vi "Dashboard Main.vi"() -> ()   [LabVIEW 2015]
uses:
  <vilib>/Utility/miscctls.llb/LVRowAndColumnTypeDef.ctl
  <vilib>/event_ctls.llb/eventvkey.ctl
  <vilib>/Rock Robotics/Network Tables/NT Read Boolean.vi
  <vilib>/Rock Robotics/WPI/Dashboard/WPI_DashboardLogging Global.vi
  <vilib>/Rock Robotics/Network Tables/NT Read Numeric Array.vi
  <vilib>/Utility/config.llb/Write Key (String).vi
  <vilib>/Utility/config.llb/Write Key (I32).vi
  <vilib>/Utility/config.llb/NI_LVConfig.lvlib
  <vilib>/vision/NI_Vision_Development_Module.lvlib
panel:
  in  "TCP":refnum<k5>
  in  "Rec Mode":enum32{"Stop", "Record", "Playback"}(radio)
  in  "Vision":u16(ring) items=["Camera Off", "USB Camera SW", "USB Camera HW", "IP Camera"]
  out "Camera IP":string
  out "Image Message":string="Timeout in Camera Communications"
  in  "Dashboard Tab":T1(tab)
  out "Camera Reversed":bool
  out "dist":dbl
  in  "Select Auto":string(combo)
  out "NT Connection":bool
  in  "Camera Settings":T2={"Frame Rate"=30, "Compression"=30, "Size"=1} {"Frame Rate" scale=1.0..30.0; "Size" items=["640x480", "320x240", "160x120"]}
  out "MotorChart R":cluster{"Numeric":dbl, "Numeric":dbl}(graph)
  out "MotorChart L":T3(graph)
  out "MotorSliders R":cluster{"MotorSlide1":dbl, "MotorSlide2":dbl} {"MotorSlide2" scale=-1.0..1.0 scale format="%#_2e"; "MotorSlide1" scale=-1.0..1.0 scale format="%#_2e"}
  out "MotorSliders L":T4 {"MotorSlide4 2" scale=0.0..14.0 scale format="%#_2e"; "MotorSlide2" scale=-1.0..1.0 scale format="%#_2e"; "MotorSlide1" scale=-1.0..1.0 scale format="%#_2e"}
  out "Gyro":dbl(knob) scale=0.0..360.0
  out "JS1 Z":dbl(slide) scale=-1.0..1.0 scale format="%#_2e"
  out "JS1 Graph":cluster{"X":dbl, "Y":dbl}[](graph)
  out "JS1 Buttons":T5
  out "JS2 Z":dbl(slide) scale=-1.0..1.0 scale format="%#_2e"
  out "JS2 Graph":cluster{"X":dbl, "Y":dbl}[](graph)
  out "JS2 Buttons":T5
  out "Mode":T6(ring)=enum."Auto Disabled"
  in  "DB Camera Config":bool
  out "fps":dbl format="%#.1g"
  out "Mbps":dbl format="%#.1g"
  out "Mbps LED":bool
  in  "DB/String 9":string
  in  "DB/String 8":string
  in  "DB/String 7":string
  in  "DB/String 6":string
  in  "DB/String 5":string
  in  "DB/String 4":string
  in  "DB/String 3":string
  in  "DB/String 2":string
  in  "DB/String 1":string
  in  "DB/String 0":string
  in  "DB/Slider 0":dbl(slide) scale=0.0..5.0
  in  "DB/Slider 1":dbl(slide) scale=0.0..5.0
  in  "DB/Slider 2":dbl(slide) scale=0.0..5.0
  in  "DB/Slider 3":dbl(slide) scale=0.0..5.0
  out "DB/LED 3":bool
  out "DB/LED 2":bool
  out "DB/LED 1":bool
  out "DB/LED 0":bool
  in  "DB/Button 3":bool
  in  "DB/Button 2":bool
  in  "DB/Button 1":bool
  in  "DB/Button 0":bool caption="New Name"
  in  "Test Slider":dbl(slide) scale=0.0..100.0 scale format="%#_3g"
  in  "On/Off":bool caption="Solenoid"
  in  "Test Name":u16(ring) items=["Select the test to run..."]
  in  "Test Tree":string(tree)
  in  "Motor":cluster{"Value":dbl, "Enable":bool} {"Value" scale=-1.0..1.0 scale format="%#_3g"}
  out "Progress":T7 {"Test Progress" scale=0.0..100.0}
  in  "Rev/Fwd":cluster{"Forward":bool, "Reverse":bool}
  in  "Test Ring":u16(ring) items=["Monochrome", "Color"]
  out "Cmd Status":string
  in  "Execute Command":bool
  in  "Command Params":string[][](table)
  in  "Command Selection":i32(listbox)
  in  "CheckList":i32(listbox)
  out "Tree":string(tree)
  out "Camera Image":T8(plugin-control)
  out "Background":bool
  # "Left"
  # "Front"
  # "Right"
  # "Battery"
  # "This tab is a great place for autonomous settings and robot-specific values.\nPlace controls and indicators inside this tab and match name to\nDashboard Variables on robot. You can also delete this comment."
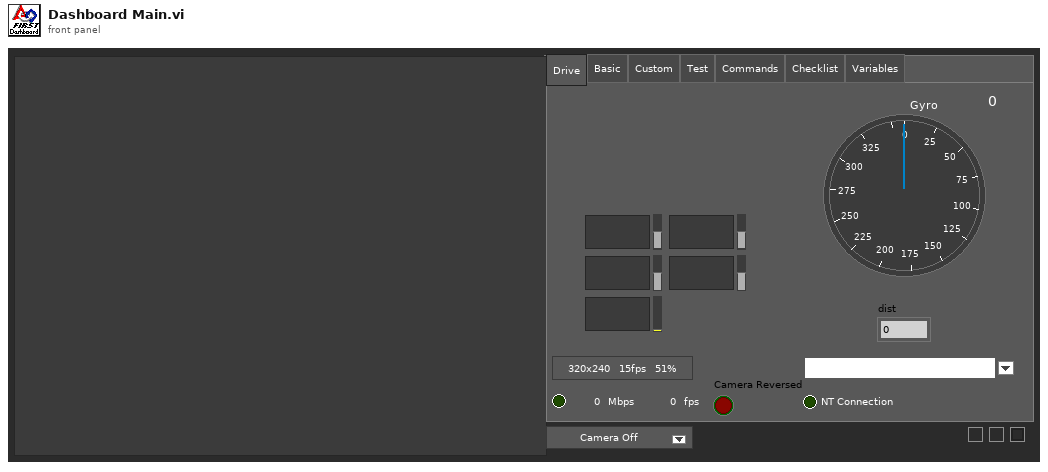
[diagram p1: front panel]
types:
  T1 = enum32{"Drive", "Basic", "Custom", "Test", "Commands", "Checklist", "Variables"}
  T2 = cluster{"Frame Rate":i32, "Compression":i32, "Size":u16}
  T3 = cluster{"Numeric":dbl, "Numeric":dbl, "Battery V":dbl}
  T4 = cluster{"MotorSlide1":dbl, "MotorSlide2":dbl, "MotorSlide4 2":dbl}
  T5 = cluster{bool, bool, bool, bool, bool, bool, bool, bool, bool, bool, bool, bool}
  T6 = enum8{"Tele-Op Disabled", "Tele-Op Enabled", "Auto Disabled", "Auto Enabled", "Test Disabled", "Test Enabled", "Disconnected", "No Code", "E-Stop"}
  T7 = cluster{"Test Progress":u8, "Test Progress Text":string}
  T8 = typedef "IMAQ Image.ctl" = refnum<image>
  T9 = cluster{"IDs":cluster{"RPC field ID":u16, "Unique ID":u16}, "String":string}
  T10 = enum32{"Drive", "Basic", "Custom", "Test", "Checklist", "Variables"}
  T11 = typedef "Image Type" = u32
  T12 = cluster{"Camera Image":refnum<vi>, "Dashboard Tab":refnum<vi>, "Background":refnum<vi>, "Vision":refnum<vi>, "Rec Mode":refnum<vi>, "Test Slider":refnum<vi>, "On/Off ":refnum<vi>, "Test Ring":refnum<vi>, "Rev/Fwd":refnum<vi>, "Test Name":refnum<vi>, "Motor":refnum<vi>, "Progress":refnum<vi>, "CheckList":refnum<vi>, "Tree":refnum<vi>, "Test Tree":refnum<vi>, "Command Params":refnum<vi>, "Command Selection":refnum<vi>, "Execute Command":refnum<vi>, "Cmd Status":refnum<vi>}
  T13 = cluster{"Error Strings":string, "Disable Counts":cluster{u16, u16}, "Rail Faults":cluster{u16, u16, u16}, "Robot IP":string, "DB Mode":u8, "Event Info":cluster{"Name":string, "Type":u8, "Number":u16, "Replay":u8}, "Camera Addr":string}
  T14 = cluster{"Storage":cluster{"Disk Free":u64, "RAM Block":u32, "RAM free":u32}, "CPU Utilization":cluster{"CPU % ISR":sgl, "CPU % Time Crit":sgl, "CPU % Timed Str":sgl, "CPU % High":sgl, "CPU % Above":sgl, "CPU % Normal":sgl, "CPU % Low":sgl}, "CAN":cluster{"% Bus Utilization":sgl, "Bus Off Cnt":u32, "TX_FIFO Full Cnt":u32, "Receive Error Cnt":u8, "Transmit Error Cnt":u8}, "HID":cluster{"HID Outputs":u32, "Rumble Low":u16, "Rumble High":u16}[]}
  T15 = cluster{"Status bits":cluster{"Test Mode":bool, "Autonomous":bool, "Enabled":bool, "Code Start":bool, "Brownout":bool, "Reserved 2":bool, "Reserved 3":bool, "E-Stop":bool}, "Code Trace":cluster{"Disabled":bool, "TeleOp":bool, "Auto":bool, "Test":bool}, "Controller Type":enum16{"unknown", "cRIO", "roboRio"}, "Code?":enum16{"unknown", "noCode", "code"}, "Battery V":dbl}
  T16 = cluster{"Control Bits":cluster{"TestMode":bool, "Autonomous":bool, "Enabled":bool, "FMS Present":bool, bool, bool, bool, "E-Stop":bool}, "Team Station ":u8, "Countdown":sgl, "Joystick Values":cluster{"Axes":dbl[], "Buttons":bool[], "POVs":i16[]}[]}
  T17 = cluster{"Axes":dbl[], "Buttons":bool[], "POVs":i16[]}[]
  T18 = cluster{"Axes":dbl[], "Buttons":bool[], "POVs":i16[]}
  T19 = cluster{"Buttons[0]":bool, "Buttons[1]":bool, "Buttons[2]":bool, "Buttons[3]":bool, "Buttons[4]":bool, "Buttons[5]":bool, "Buttons[6]":bool, "Buttons[7]":bool, "Buttons[8]":bool, "Buttons[9]":bool, "Buttons[10]":bool, "Buttons[11]":bool}
  T20 = typedef "NI_LVConfig.lvlib/Config Data RefNum.ctl" = refnum<k1>
  T21 = cluster{"Operation":enum16{"Update", "Clear"}, "Color Box":u32}[]
  T22 = typedef "eventvkey.ctl" = enum16{"ASCII", "Enter", "Return", "Shift", "Ctrl", "Alt", "Cmd", "Opt", "Caps", "NumLock", "Clear", "Break", "Up", "Down", "Left", "Right", "Insert", "Delete", "Home", "End", "PageUp", "PageDown", "Escape", "Help", "Pause", "ScrollLock", "F1", "F2", "F3", "F4", "F5", "F6", "F7", "F8", "F9", "F10", "F11", "F12", "F13", "F14", "F15", "F16", "F17", "F18", "F19", "F20", "F21", "F22", "F23", "F24", "Play", "VolumeUp", "VolumeDown", "Mute", "Two Byte Char"}
  T23 = cluster{"Image Size":bool, "Image Type":bool, "Pixel Value":bool, "ROI Information":bool, "Zoom Factor":bool}
  T24 = enum8{"Enabled", "Disabled", "Disabled and Grayed Out"}
  T25 = cluster{"Operation":enum16{"Update", "Clear"}, "Color Box":u32}
  T26 = typedef "LVRowAndColumnTypeDef.ctl" = cluster{"Row":i32, "Column":i32}
  T27 = cluster{"Shift":bool, "Ctrl":bool, "Alt":bool, "Cmd":bool, "Opt":bool}
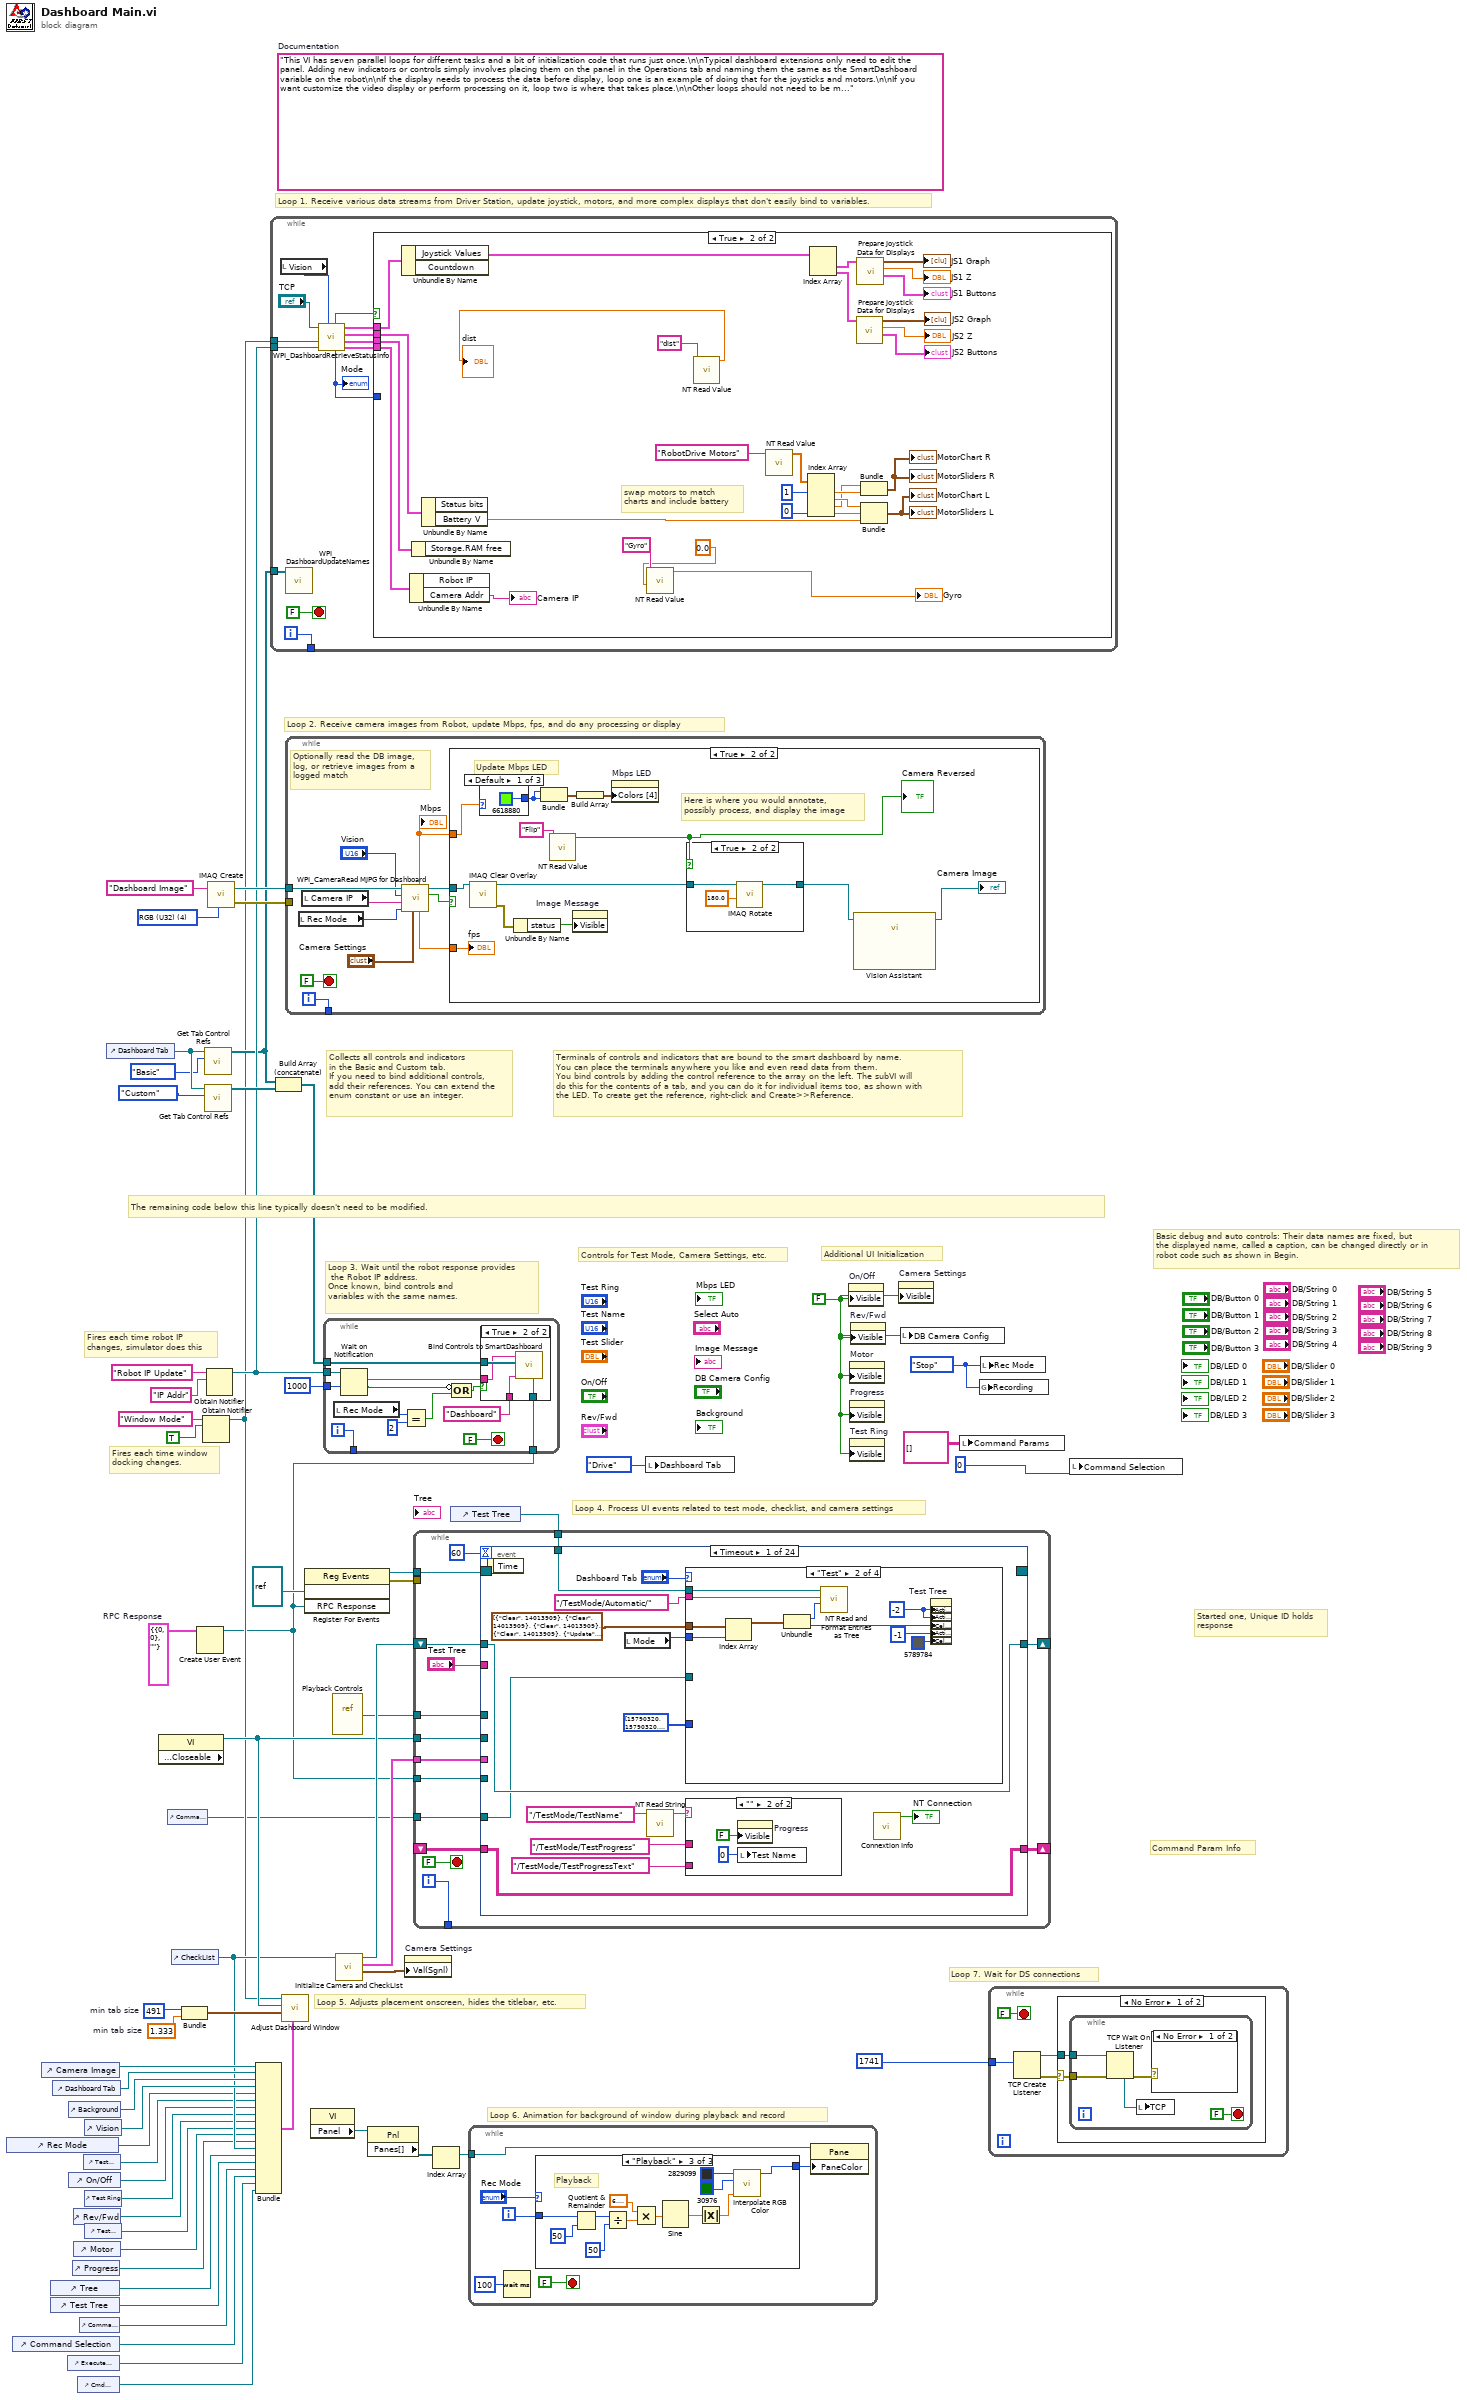
[diagram p0: block diagram]
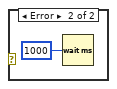
[diagram p2: hidden frame]
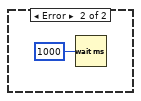
[diagram p3: hidden frame]
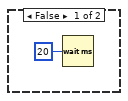
[diagram p4: hidden frame]
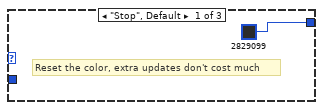
[diagram p5: hidden frame]
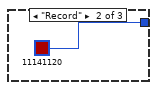
[diagram p6: hidden frame]
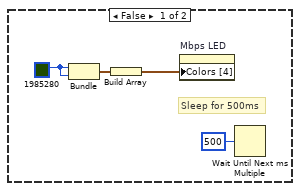
[diagram p8: hidden frame]
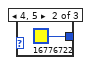
[diagram p10: hidden frame]
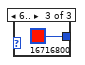
[diagram p11: hidden frame]
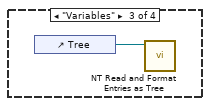
[diagram p13: hidden frame]
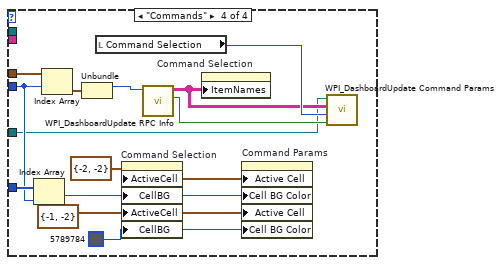
[diagram p14: hidden frame]
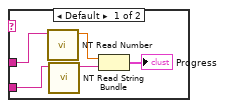
[diagram p15: hidden frame]
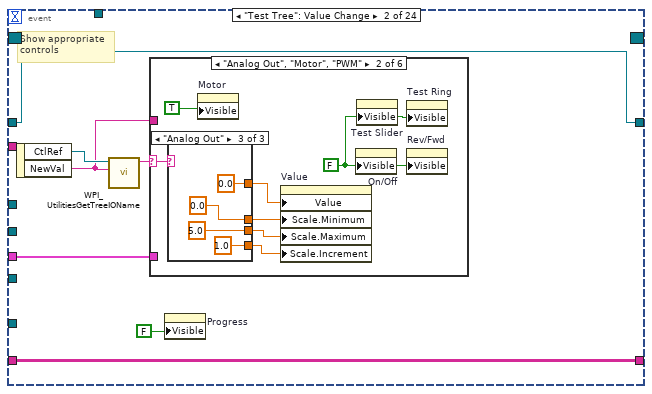
[diagram p16: hidden frame]
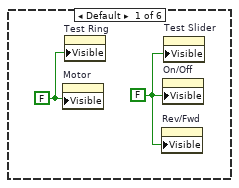
[diagram p17: hidden frame]
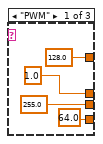
[diagram p18: hidden frame]
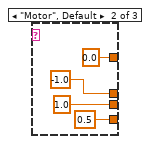
[diagram p19: hidden frame]
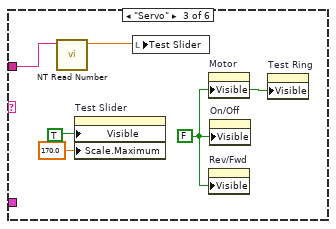
[diagram p20: hidden frame]
diagram:
  w7 = T9 {"IDs"={"RPC field ID"=0, "Unique ID"=0}, "String"=""}  # RPC Response
  w33 = 491  # min tab size
  w32 = 1.333  # min tab size
  w41 = enum32{"Stop", "Record", "Playback"}."Stop" ("Rec Mode")
  w15 = FALSE ("Visible")
  (unwired) "This VI has seven parallel loops for different tasks and a bit of initialization code that runs just once.\n\nTypical dashboard extensions only need to edit the panel. Adding new indicators or controls simply involves placing them on the panel in the Operations tab and naming them the same as the SmartDashboard variable on the robot\n\nIf the display needs to process the data before display, loop one is an example of doing that for the joysticks and motors.\n\nIf you want customize the video display or perform processing on it, loop two is where that takes place.\n\nOther loops should not need to be modified. They are pretty standard, and document the task they perform."  # Documentation
  w61 = T11 4 items=["Grayscale (U8)", "Grayscale (I16)", "Grayscale (SGL)", "Complex (CSG)", "RGB (U32)", "HSL (U32)", "RGB (U64)"] ("Image Type")
  # "Command Param Info"
  # "Started one, Unique ID holds\nresponse"
  # "Loop 7. Wait for DS connections"
  # "Basic debug and auto controls: Their data names are fixed, but\nthe displayed name, called a caption, can be changed directly or in\nrobot code such as shown in Begin."
  # "Controls for Test Mode, Camera Settings, etc."
  # "Additional UI Initialization"
  # "Loop 6. Animation for background of window during playback and record"
  # "Fires each time robot IP\nchanges, simulator does this"
  # "Fires each time window\ndocking changes."
  # "Collects all controls and indicators\nin the Basic and Custom tab.\nIf you need to bind additional controls,\nadd their references. You can extend the\nenum constant or use an integer."
  # "The remaining code below this line typically doesn't need to be modified."
  # "Loop 4. Process UI events related to test mode, checklist, and camera settings"
  # "Terminals of controls and indicators that are bound to the smart dashboard by name.\nYou can place the terminals anywhere you like and even read data from them.\nYou bind controls by adding the control reference to the array on the left. The subVI will\ndo this for the contents of a tab, and you can do it for individual items too, as shown with\nthe LED. To create get the reference, right-click and Create>>Reference."
  # "Loop 3. Wait until the robot response provides\n the Robot IP address.\nOnce known, bind controls and\nvariables with the same names."
  # "Loop 5. Adjusts placement onscreen, hides the titlebar, etc."
  # "Loop 1. Receive various data streams from Driver Station, update joystick, motors, and more complex displays that don't easily bind to variables."
  # "Loop 2. Receive camera images from Robot, update Mbps, fps, and do any processing or display"
  n1 = control-ref of="Rec Mode"() -> (w21:refnum<vi>)
  n2 = control-ref of="Command Selection"() -> (w6:refnum<vi>)
  n3 = control-ref of="Camera Image"() -> (w36:refnum<vi>)
  n4 = control-ref of="Tree"() -> (w25:refnum<vi>)
  n5 = control-ref of="Test Tree"() -> (w24:refnum<vi>)
  n6 = control-ref of="Dashboard Tab"() -> (w35:refnum<vi>)
  n7 = control-ref of="Execute Command"() -> (w8:refnum<vi>)
  n8 = control-ref of="Background"() -> (w30:refnum<vi>)
  n9 = control-ref of="On/Off"() -> (w19:refnum<vi>)
  n10 = control-ref of="Progress"() -> (w16:refnum<vi>)
  n11 = control-ref of="Rev/Fwd"() -> (w17:refnum<vi>)
  n12 = control-ref of="Motor"() -> (w22:refnum<vi>)
  n13 = control-ref of="Cmd Status"() -> (w2:refnum<vi>)
  n14 = control-ref of="Command Params"() -> (w9:refnum<vi>)
  n15 = control-ref of="Test Slider"() -> (w20:refnum<vi>)
  n16 = control-ref of="Vision"() -> (w34:refnum<vi>)
  n17 = control-ref of="Test Ring"() -> (w18:refnum<vi>)
  n18 = control-ref of="Test Name"() -> (w23:refnum<vi>)
  n19 = control-ref of="Dashboard Tab"() -> (w39:refnum<vi>)
  n20 = property class="VI" props=["Front Panel.Closeable"]() -> (reference out=w40:refnum<vi>)  [unwired: 2 in, 2 out]
  n21 = control-ref of="Command Params"() -> (w1:refnum<vi>)
  n22 = control-ref of="CheckList"() -> (w26:refnum<vi>)
  n23 = Bundle("min tab size"=w33, "min tab size"=w32) -> (w31:cluster{"min tab size":i32, "min tab size":dbl})  [unwired: 1 in]
  n24 = Create User Event(user event datatype=w7) -> (user event=w3:refnum<user-event>)  [unwired: 1 in, 1 out]
  n25 = Obtain Notifier(name (unnamed)="Window Mode", notification data type=TRUE) -> (notifier out=w12:refnum<notifier>)  [unwired: 2 in, 2 out]
  n26 = call <vilib>:"Get Tab Control Refs.vi"("Page Index"=T10."Basic" ("Dashboard Tab"), "TabControl in"=w39) -> ("ControlsOnPage"=w13:refnum<vi>[])  [unwired: 9 in]
  n27 = call <vilib>:"Get Tab Control Refs.vi"("Page Index"=T10."Custom" ("Dashboard Tab"), "TabControl in"=w39) -> ("ControlsOnPage"=w38:refnum<vi>[])  [unwired: 9 in]
  n28 = Obtain Notifier(name (unnamed)="Robot IP Update", notification data type="IP Addr" ("name (unnamed)")) -> (notifier out=w14:refnum<notifier>)  [unwired: 2 in, 2 out]
  n29 = call "IMAQ Create"("Image Name"="Dashboard Image", "Image Type"=w61) -> ("New Image"=w59:T8, "error out"=w58:errorcluster)  [unwired: 2 in, 1 out]
  n30 = Bundle("Camera Image"=w36, "Dashboard Tab"=w35, "Background"=w30, "Vision"=w34, "Rec Mode"=w21, "Test Slider"=w20, "On/Off"=w19, "Test Ring"=w18, "Rev/Fwd"=w17, "Test Name"=w23, "Motor"=w22, "Progress"=w16, "CheckList"=w26, "Tree"=w25, "Test Tree"=w24, "Command Params"=w9, "Command Selection"=w6, "Execute Command"=w8, "Cmd Status"=w2) -> (w27:T12)  [unwired: 1 in]
  n31 = while {
    tunnel: [w73] -> _
    tunnel: w14 -> [w67]
    tunnel: w13 -> [w66]
    tunnel: w12 -> [w62]
    i -> [w73]
    stop <- FALSE stop-if-true
    n32 = local read "Vision"() -> (w64:u16)
    n33 = call <vilib>:"WPI_DashboardUpdateNames.vi"("Controls on Tab"=w66) -> ()  [unwired: 11 in]
    n34 = call <vilib>:"WPI_DashboardRetrieveStatusInfo.vi"("Vision"=w64, "Binding Refnum"=w67, "Window Mode Notifier"=w62, "TCP Cnx"="TCP") -> ("Power and Errors"=w68:T13, "Robot Metrics"=w71:T14, "Status Info"=w72:T15, "Control Info"=w69:T16, "Robot Mode"=w65:T6, "Process?"=w70:bool)  [unwired: 2 in]
    "Mode" <- w65
    n35 = case shown="True" w70 {
      tunnel: w72 -> [_ w105]
      tunnel: w71 -> [_ w104]
      tunnel: w69 -> [_ w103]
      tunnel: w68 -> [_ w102]
      tunnel: w65 -> [_ _]
      frame False {
        n36 = Wait (ms)(milliseconds to wait=u32 20) -> ()  [unwired: 1 out]
      }
      frame True {
        # "swap motors to match\ncharts and include battery"
        n37 = Unbundle By Name(w103) -> ("Joystick Values"=w92:T17)  [unwired: 1 out]
        n38 = Unbundle By Name(w102) -> ("Camera Addr"=→"Camera IP":string)  [unwired: 1 out]
        n39 = Unbundle By Name(w104) -> ()  [unwired: 1 out]
        n40 = Unbundle By Name(w105) -> ("Battery V"=w93:dbl)  [unwired: 1 out]
        n41 = call-poly <vilib>:"NT Read Value.vi"("Default Value"=0.0 ("y"), "Name"="Gyro") -> ("Numeric"=→"Gyro":dbl)  [unwired: 8 in, 1 out]
        n42 = call-poly <vilib>:"NT Read Value.vi"("Name"="dist") -> ("Numeric"=→"dist":dbl)  [unwired: 9 in, 1 out]
        n43 = call-poly <vilib>:"NT Read Value.vi"("Name"="RobotDrive Motors") -> ("Numeric Array"=w81:dbl[])  [unwired: 9 in, 1 out]
        n44 = Index Array(array=w81, index #1=1, index #4=0) -> (element #1=w97:dbl, element #2=w98:dbl, element #3=w96:dbl, element #4=w101:dbl)  [unwired: 2 in]
        n45 = Index Array(array=w92) -> (element #1=w91:T18, element #2=w86:T18)  [unwired: 2 in]
        n46 = call "Prepare Joystick Data for Displays.vi"("Joystick Values"=w86) -> ("Buttons"=→"JS2 Buttons":T19, "Z Axis"=→"JS2 Z":dbl, "Cartesian Data"=→"JS2 Graph":cluster{"X axis":dbl, "X axis":dbl}[])  [unwired: 8 in]
        n47 = call "Prepare Joystick Data for Displays.vi"("Joystick Values"=w91) -> ("Buttons"=→"JS1 Buttons":T19, "Z Axis"=→"JS1 Z":dbl, "Cartesian Data"=→"JS1 Graph":cluster{"X axis":dbl, "X axis":dbl}[])  [unwired: 8 in]
        n48 = Bundle("Numeric"=w96, "Numeric"=w97) -> (→"MotorChart R" →"MotorSliders R":cluster{"Numeric":dbl, "Numeric":dbl})  [unwired: 1 in]
        n49 = Bundle("Numeric"=w98, "Numeric"=w101, "Battery V"=w93) -> (→"MotorChart L" →"MotorSliders L":T3)  [unwired: 1 in]
      }
    }
  }
  n50 = Build Array (concatenate)(w13, w38) -> (w37:refnum<vi>[])
  n51 = call "Adjust Dashboard Window.vi"("Sizing Refnums"=w27, "Size Constraints"=w31, "VI"=w40, "WIn Mode"=w12) -> ()  [unwired: 8 in]
  n52 = while {
    tunnel: w59 -> [w114]
    tunnel: w58 -> [_]
    tunnel: [w115] -> _
    i -> [w115]
    stop <- FALSE stop-if-true
    # "Optionally read the DB image,\nlog, or retrieve images from a\nlogged match"
    n53 = local read "Rec Mode"() -> (w109:enum32{"Stop", "Record", "Playback"})
    n54 = local read "Camera IP"() -> (w107:string)
    n55 = call <vilib>:"WPI_CameraRead MJPG for Dashboard.vi"("Camera Settings"="Camera Settings", "Rec Mode"=w109, "Camera IP"=w107, "Camera Mode"="Vision", "Refnum in"=w114) -> ("Active"=w112:bool, "Refnum out"=w113:T8, "FPS"=w111:dbl, "Bandwidth (Mbps)"=w106:dbl)  [unwired: 3 in]
    "Mbps" <- w106
    n56 = case shown="True" w112 {
      tunnel: w113 -> [_ w128]
      tunnel: w106 -> [_ w127]
      tunnel: w111 -> [_ w126]
      frame False {
        w117 = u32 1985280 ("Color Box")
        # "Sleep for 500ms"
        n57 = Bundle("Color Box"=w117, "Color Box"=w117) -> (w119:cluster{"Color Box":u32, "Color Box":u32})  [unwired: 1 out]
        n58 = Build Array(w119) -> (w118:cluster{"Color Box":u32, "Color Box":u32}[])
        n59 = property on="Mbps LED" class="Bool (strict)"("Colors [4]"=w118) -> ()  [unwired: 2 in, 2 out]
        n60 = Wait Until Next ms Multiple(millisecond multiple=u32 500) -> ()  [unwired: 1 out]
      }
      frame True {
        # "Here is where you would annotate,\npossibly process, and display the image"
        # "Update Mbps LED"
        n61 = call "IMAQ Clear Overlay"("Image"=w128) -> ("error out"=w132:errorcluster, "Image Out"=w125:T8)  [unwired: 2 in, 7 out]
        n62 = case shown="Default" w127 {
          tunnel: [u32 6618880 ("Color Box") u32 16776722 ("Color Box") u32 16716800 ("Color Box")] -> w129
          frame Default {
          }
          frame 4, 5 {
          }
          frame 6.. {
          }
        }
        n63 = Unbundle By Name(w132) -> ("status"=w133:bool)
        n64 = Bundle("Color Box"=w129, "Color Box"=w129) -> (w131:cluster{"Color Box":u32, "Color Box":u32})  [unwired: 1 out]
        n65 = call-poly <vilib>:"NT Read Value.vi"("Name"="Flip") -> ("Boolean"=w123:bool)  [unwired: 9 in, 1 out]
        "Camera Reversed" <- w123
        n66 = property on="Image Message" class="Str"("Visible"=w133) -> ()  [unwired: 2 in, 2 out]
        n67 = Build Array(w131) -> (w130:cluster{"Color Box":u32, "Color Box":u32}[])
        n68 = property on="Mbps LED" class="Bool (strict)"("Colors [4]"=w130) -> ()  [unwired: 2 in, 2 out]
        n69 = case shown="True" w123 {
          tunnel: w125 -> [w134 w137]
          tunnel: [w134 w136] -> w122
          frame False {
          }
          frame True {
            n70 = call "IMAQ Rotate"("Angle (degrees)"=sgl 180.0, "Image Src"=w137) -> ("Image Dst Out"=w136:T8)  [unwired: 8 in, 1 out]
          }
        }
        n71 = call "Vision Assistant"("Image In"=w122) -> ("Image Out"=→"Camera Image":T8)  [unwired: 25 in, 1 out]
        "fps" <- w126
      }
    }
  }
  n72 = register-events(refnum<vi> refnum, w3) -> (reference out=w45:refnum<event-registration>, error out=w44:errorcluster)  [unwired: 2 in]
  n73 = property class="VI"() -> ("Panel"=w48:refnum<vi>)  [unwired: 2 in, 2 out]
  n74 = while {
    tunnel: w37 -> [w153]
    tunnel: w14 -> [w151]
    tunnel: [w149] -> _
    tunnel: u32 1000 ("milliseconds to wait") -> [w148]
    tunnel: w3 -> [w141]
    i -> [w149]
    stop <- FALSE stop-if-true
    n75 = local read "Rec Mode"() -> (w144:enum32{"Stop", "Record", "Playback"})
    n76 = Wait on Notification(notifier=w151, timeout in ms (-1)=w148) -> (notification=w150:string, timed out?=w146:bool)  [unwired: 2 in, 2 out]
    n77 = Equal?(x=w144, y=u16 2 ("Rec Mode")) -> (x = y?=w145:bool)
    n78 = Compound Arithmetic op=OR(invert w146, w145) -> (w147:bool)
    n79 = case shown="True" w147 {
      tunnel: w153 -> [_ w157]
      tunnel: w150 -> [_ w156]
      tunnel: "Dashboard" -> [_ w155]
      tunnel: w141 -> [_ w154]
      frame False {
      }
      frame True {
        n80 = call <vilib>:"Bind Controls to SmartDashboard.vi"("RPC ref"=w154, "Client Name"=w155, "Bound Control Refs"=w157, "Server IP Address"=w156) -> ()  [unwired: 8 in]
      }
    }
  }
  n81 = vi-ref "Playback Controls.vi"() -> (w46:refnum<vi>)
  n82 = call "Initialize Camera and CheckList.vi"("ListBox in"=w26) -> ("Cluster"=w52:cluster{"value":i32, "value":i32, "index":i32}, "Array"=w53:cluster{string[]}[], "File Refnum"=w51:T20)  [unwired: 8 in]
  n83 = property class="Pnl"(reference=w48) -> ("Panes[]"=w49:refnum<vi>[])  [unwired: 1 in, 2 out]
  n84 = property on="Camera Settings" class="Clust (strict)"("Val(Sgnl)"=w52) -> ()  [unwired: 2 in, 2 out]
  n85 = Index Array(array=w49) -> (element=w47:refnum<vi>)  [unwired: 1 in]
  n86 = control-ref of="Test Tree"() -> (w50:refnum<vi>)
  n87 = while {
    tunnel: w53 -> [w169]
    shift-right: [w168] -> _
    shift-left: w51 -> [w167]
    tunnel: [w166] -> _
    tunnel: w50 -> [w165]
    tunnel: w46 -> [w164]
    tunnel: w45 -> [w163]
    tunnel: w44 -> [_]
    tunnel: w40 -> [w162]
    tunnel: w3 -> [w161]
    tunnel: w1 -> [w160]
    shift-right: [w159] -> _
    shift-left: _ -> [w158]
    i -> [w166]
    stop <- FALSE stop-if-true
    n88 = event shown="[0] Timeout" {
      selector: w163 -> [_ _ _ _ _ _ _ _ _ _ _ _ _ _ _ _ _ _ _ _ _ _ _ _]
      dyn-events: [_ _ _ _ _ _ _ _ _ _ _ _ _ _ _ _ _ _ w478 _ _ _ _ _] -> _
      timeout: u32 60 ("milliseconds to wait") -> [_ _ _ _ _ _ _ _ _ _ _ _ _ _ _ _ _ _ _ _ _ _ _ _]
      tunnel: w165 -> [w182 _ _ _ _ _ _ _ _ _ _ _ _ _ _ _ _ _ _ _ _ _ _ _]
      tunnel: "Test Tree" -> [_ _ _ _ _ _ _ _ _ _ _ _ _ w441 w450 w453 w458 w467 _ _ _ _ _ _]
      tunnel: w169 -> [_ w220 _ _ _ _ _ _ _ _ _ w403 w434 _ _ _ _ _ _ _ _ _ _ _]
      tunnel: [w179 w219 w323 w329 w339 w343 w349 w361 w369 w375 w388 w402 w427 w440 w448 w452 w457 w466 w480 w496 w498 w506 w517 w522] -> w168
      tunnel: w167 -> [w179 w219 w323 w329 w339 w343 w349 w361 w369 w375 w388 w401 w427 w440 w448 w452 w457 w466 w480 w496 w498 w506 w517 w522]
      tunnel: w164 -> [_ _ _ _ _ _ _ _ _ _ _ _ _ _ _ _ _ _ w481 _ w501 _ _ _]
      tunnel: w162 -> [_ _ _ _ _ _ _ _ _ _ _ _ _ _ _ _ _ _ w476 _ _ _ _ _]
      tunnel: w161 -> [_ _ _ _ _ _ _ _ _ _ _ _ _ _ _ _ _ _ w472 _ _ _ _ _]
      tunnel: w160 -> [w174 _ _ _ _ _ w347 _ _ _ _ _ _ _ _ _ _ _ _ _ _ _ _ _]
      tunnel: [w173 w218 w322 w328 w338 w344 w345 w355 w366 w374 w387 w400 w426 w439 w447 w451 w456 w465 w471 w494 w497 w502 w510 w523] -> w159
      tunnel: w158 -> [w173 w218 w322 w328 w338 w344 w345 _ _ w374 w387 w400 w426 w439 w447 w451 w456 w465 w471 w494 w497 w502 w510 w523]
      event Timeout {
        n89 = event-data() -> ()  [unwired: 1 in, 1 out]
        n90 = local read "Mode"() -> (w176:T6)
        n91 = call <vilib>:"NT Read String.vi"("Name"="/TestMode/TestName") -> ("String"=w185:string)  [unwired: 9 in, 1 out]
        n92 = case shown="\"Test\"" "Dashboard Tab" {
          tunnel: w182 -> [_ w196 _ _]
          tunnel: "/TestMode/Automatic/" ("Name Pattern") -> [_ w195 _ _]
          tunnel: T21 [{"Operation"=enum."Clear", "Color Box"=14013909}, {"Operation"=enum."Clear", "Color Box"=14013909}, {"Operation"=enum."Clear", "Color Box"=14013909}, {"Operation"=enum."Clear", "Color Box"=14013909}, {"Operation"=enum."Update", "Color Box"=14013909}, {"Operation"=enum."Update", "Color Box"=16777215}, {"Operation"=enum."Clear", "Color Box"=14013909}, {"Operation"=enum."Clear", "Color Box"=14013909}, {"Operation"=enum."Clear", "Color Box"=14013909}] -> [_ w188 _ w205]
          tunnel: w176 -> [_ w187 _ w204]
          tunnel: u32[] [15790320, 15790320, 15790320, 15790320, 16777215, 16777215, 15790320, 15790320, 15790320] -> [_ _ _ w210]
          tunnel: w174 -> [_ _ _ w198]
          frame "Custom", Default {
          }
          frame "Test" {
            w194 = -2 ("Active Item:Row Number")
            n93 = Index Array(array=w188, index=w187) -> (element=w189:T25)
            n94 = Unbundle(w189) -> ("Operation"=w190:enum16{"Update", "Clear"}, "Color Box"=w191:u32)
            n95 = call <vilib>:"NT Read and Format Entries as Tree.vi"("Operation"=w190, "Name Pattern"=w195, "Tree Refnum"=w196) -> ()  [unwired: 7 in, 2 out]
            n96 = property on="Test Tree" class="Tree (strict)"("Active Item Row Number"=w194, "ActiveColNum"=w194, "CellBG"=w191, "Active Item Row Number"=-1 ("Active Item:Row Number"), "CellBG"=u32 5789784 ("Color Box")) -> ()  [unwired: 2 in, 2 out]
          }
          frame "Variables" {
            n97 = control-ref of="Tree"() -> (w197:refnum<vi>)
            n98 = call <vilib>:"NT Read and Format Entries as Tree.vi"("Tree Refnum"=w197) -> ()  [unwired: 9 in, 2 out]
          }
          frame "Commands" {
            w206 = u32 5789784 ("Color Box")
            w207 = T26 {"Row"=-1, "Column"=-2} ("Active Cell:Active Cell")
            w209 = T26 {"Row"=-2, "Column"=-2} ("Active Cell:Active Cell")
            n99 = Index Array(array=w210, index=w204) -> (element=w208:u32)
            n100 = Index Array(array=w205, index=w204) -> (element=w203:T25)
            n101 = Unbundle(w203) -> ("Operation"=w202:enum16{"Update", "Clear"})  [unwired: 1 out]
            n102 = local read "Command Selection"() -> (w201:i32)
            n103 = property on="Command Selection" class="MCListbox (strict)"("ActiveCell"=w209, "CellBG"=w208, "ActiveCell"=w207, "CellBG"=w206) -> ()  [unwired: 2 in, 2 out]
            n104 = call <vilib>:"WPI_DashboardUpdate RPC Info.vi"("Operation"=w202) -> ("update"=w200:bool, "commands"=w199:string[][])  [unwired: 9 in]
            n105 = property on="Command Selection" class="MCListbox (strict)"("ItemNames"=w199) -> ()  [unwired: 2 in, 2 out]
            n106 = property on="Command Params" class="Tbl (strict)"("Active Cell"=w209, "Cell BG Color"=w208, "Active Cell"=w207, "Cell BG Color"=w206) -> ()  [unwired: 2 in, 2 out]
            n107 = call <vilib>:"WPI_DashboardUpdate Command Params.vi"("Update"=w200, "NewVal"=w201, "Commands"=w199, "Param Tbl"=w198) -> ()  [unwired: 7 in, 1 out]
          }
        }
        n108 = case shown="\"\"" w185 {
          tunnel: "/TestMode/TestProgress" ("Name") -> [w212 _]
          tunnel: "/TestMode/TestProgressText" ("Name") -> [w211 _]
          frame Default {
            n109 = call <vilib>:"NT Read Number.vi"("Name"=w212) -> ("Numeric"=w213:dbl)  [unwired: 9 in, 1 out]
            n110 = call <vilib>:"NT Read String.vi"("Name"=w211) -> ("String"=w214:string)  [unwired: 9 in, 1 out]
            n111 = Bundle("Numeric"=w213, "String"=w214) -> (→"Progress":cluster{"Numeric":dbl, "String":string})  [unwired: 1 in]
          }
          frame "" {
            n112 = property on="Progress" class="Clust (strict)"("Visible"=FALSE) -> ()  [unwired: 2 in, 2 out]
            n113 = local write "Test Name"(u16 0) -> ()
          }
        }
        n114 = call <vilib>:"Connextion Info.vi"() -> ("Connected"=→"NT Connection":bool)  [unwired: 10 in, 1 out]
      }
      event "Test Tree": Value Change {
        # "Show appropriate\ncontrols"
        n115 = event-data() -> ("CtlRef"=w223:refnum<vi>, "NewVal"=w221:string)  [unwired: 1 in]
        n116 = call <vilib>:"WPI_UtilitiesGetTreeIOName.vi"("NewVal"=w221, "TreeControl in"=w223) -> ("I/O Name"=w224:string)  [unwired: 9 in]
        n117 = case shown="\"Analog Out\", \"Motor\", \"PWM\"" w224 {
          selector: w224 -> [_ w231 _ w253 w262 _]
          tunnel: w221 -> [_ _ w250 w252 _ w269]
          tunnel: w220 -> [_ _ _ _ _ w268]
          frame Default {
            w226 = FALSE ("Visible")
            w225 = FALSE ("Visible")
            n118 = property on="Motor" class="Clust (strict)"("Visible"=w225) -> ()  [unwired: 2 in, 2 out]
            n119 = property on="Test Ring" class="Ring (strict)"("Visible"=w225) -> ()  [unwired: 2 in, 2 out]
            n120 = property on="Rev/Fwd" class="Clust (strict)"("Visible"=w226) -> ()  [unwired: 2 in, 2 out]
            n121 = property on="On/Off" class="Bool (strict)"("Visible"=w226) -> ()  [unwired: 2 in, 2 out]
            n122 = property on="Test Slider" class="Slide (strict)"("Visible"=w226) -> ()  [unwired: 2 in, 2 out]
          }
          frame "Analog Out", "Motor", "PWM" {
            w232 = FALSE ("Visible")
            n123 = case shown="\"Analog Out\"" w231 {
              tunnel: [1.0 ("Value") -1.0 ("Value") 0.0 ("Value")] -> w230
              tunnel: [255.0 ("Value") 1.0 ("Value") 5.0 ("Value")] -> w229
              tunnel: [128.0 ("Value") 0.0 ("Value") 0.0 ("Value")] -> w228
              tunnel: [64.0 ("Value") 0.5 ("Value") 1.0 ("Value")] -> w227
              frame "PWM" {
              }
              frame "Motor", Default {
              }
              frame "Analog Out" {
              }
            }
            n124 = property on="Motor" class="Clust (strict)"("Visible"=TRUE) -> ()  [unwired: 2 in, 2 out]
            n125 = property on="Value" class="Slide (strict)"("Value"=w228, "Scale.Minimum"=w230, "Scale.Maximum"=w229, "Scale.Increment"=w227) -> ()  [unwired: 2 in, 2 out]
            n126 = property on="On/Off" class="Bool (strict)"("Visible"=w232) -> ()  [unwired: 2 in, 2 out]
            n127 = property on="Test Slider" class="Slide (strict)"("Visible"=w232) -> ()  [unwired: 2 in, 2 out]
            n128 = property on="Test Ring" class="Ring (strict)"("Visible"=w232) -> ()  [unwired: 2 in, 2 out]
            n129 = property on="Rev/Fwd" class="Clust (strict)"("Visible"=w232) -> ()  [unwired: 2 in, 2 out]
          }
          frame "Servo" {
            w248 = FALSE ("Visible")
            n130 = call <vilib>:"NT Read Number.vi"("Name"=w250) -> ("Numeric"=w249:dbl)  [unwired: 9 in, 1 out]
            n131 = property on="Test Slider" class="Slide (strict)"("Visible"=TRUE, "Scale.Maximum"=170.0 ("Scale.Range:Maximum")) -> ()  [unwired: 2 in, 2 out]
            n132 = local write "Test Slider"(w249) -> ()
            n133 = property on="Motor" class="Clust (strict)"("Visible"=w248) -> ()  [unwired: 2 in, 2 out]
            n134 = property on="Rev/Fwd" class="Clust (strict)"("Visible"=w248) -> ()  [unwired: 2 in, 2 out]
            n135 = property on="On/Off" class="Bool (strict)"("Visible"=w248) -> ()  [unwired: 2 in, 2 out]
            n136 = property on="Test Ring" class="Ring (strict)"("Visible"=w248) -> ()  [unwired: 2 in, 2 out]
          }
          frame "Relay", "Solenoid" {
            w251 = FALSE ("Visible")
            n137 = property on="Motor" class="Clust (strict)"("Visible"=w251) -> ()  [unwired: 2 in, 2 out]
            n138 = property on="Test Slider" class="Slide (strict)"("Visible"=w251) -> ()  [unwired: 2 in, 2 out]
            n139 = Search and Replace String(input string=w252, search string="/Value  **", replace string="/Direction") -> (result string=w258:string)  [unwired: 5 in, 3 out]
            n140 = property on="Test Ring" class="Ring (strict)"("Visible"=w251) -> ()  [unwired: 2 in, 2 out]
            n141 = call <vilib>:"NT Read String.vi"("Name"=w258) -> ("String"=w256:string)  [unwired: 9 in, 1 out]
            n142 = Equal?(x="Both directions", y=w256) -> (x = y?=w254:bool)
            n143 = Not(x=w254) -> (.not. x?=w255:bool)
            n144 = property on="Rev/Fwd" class="Clust (strict)"("Visible"=w254) -> ()  [unwired: 2 in, 2 out]
            n145 = property on="On/Off" class="Bool (strict)"("Visible"=w255, "Caption.Text"=w253) -> ()  [unwired: 2 in, 2 out]
          }
          frame "Compressor", "Digital Out" {
            w261 = FALSE ("Visible")
            # "Get direction and finish"
            n146 = property on="Motor" class="Clust (strict)"("Visible"=w261) -> ()  [unwired: 2 in, 2 out]
            n147 = property on="Test Slider" class="Slide (strict)"("Visible"=w261) -> ()  [unwired: 2 in, 2 out]
            n148 = property on="Test Ring" class="Ring (strict)"("Visible"=w261) -> ()  [unwired: 2 in, 2 out]
            n149 = property on="On/Off" class="Bool (strict)"("Visible"=TRUE, "Caption.Text"=w262) -> ()  [unwired: 2 in, 2 out]
            n150 = property on="Rev/Fwd" class="Clust (strict)"("Visible"=FALSE) -> ()  [unwired: 2 in, 2 out]
          }
          frame "Camera" {
            n151 = call <vilib>:"Get Last Path Segment.vi"("String in"=w269) -> ("String out"=w270:string)  [unwired: 10 in]
            n152 = property on="On/Off" class="Bool (strict)"("Visible"=FALSE) -> ()  [unwired: 2 in, 2 out]
            n153 = property on="Motor" class="Clust (strict)"("Visible"=FALSE) -> ()  [unwired: 2 in, 2 out]
            n154 = property on="Rev/Fwd" class="Clust (strict)"("Visible"=FALSE) -> ()  [unwired: 2 in, 2 out]
            n155 = case shown="\"White Balance  **\"" w270 {
              tunnel: w269 -> [w276 w285 w294 w303 w312 _ w318]
              tunnel: w268 -> [w274 w282 w291 w300 w309 _ _]
              frame "Size  **" {
                n156 = Index Array(array=w274) -> (element=w273:cluster{string[]})  [unwired: 1 in]
                n157 = call <vilib>:"NT Read String.vi"("Name"=w276) -> ("String"=w275:string)  [unwired: 9 in, 1 out]
                n158 = Unbundle(w273) -> (w271:string[])
                n159 = Match First String(2:w271, 3:w275) -> (0:w272:i32)  [unwired: 1 out]
                n160 = property on="Test Ring" class="Ring (strict)"("Value"=w272, "Strings []"=w271) -> ()  [unwired: 2 in, 2 out]
                n161 = property on="Test Ring" class="Ring (strict)"("Visible"=TRUE) -> ()  [unwired: 2 in, 2 out]
                n162 = property on="Test Slider" class="Slide (strict)"("Visible"=FALSE) -> ()  [unwired: 2 in, 2 out]
              }
              frame "White Balance  **" {
                n163 = Index Array(array=w282, index=1) -> (element=w283:cluster{string[]})
                n164 = call <vilib>:"NT Read String.vi"("Name"=w285) -> ("String"=w284:string)  [unwired: 9 in, 1 out]
                n165 = Unbundle(w283) -> (w280:string[])
                n166 = Match First String(2:w280, 3:w284) -> (0:w279:i32)  [unwired: 1 out]
                n167 = property on="Test Ring" class="Ring (strict)"("Value"=w279, "Strings []"=w280) -> ()  [unwired: 2 in, 2 out]
                n168 = property on="Test Ring" class="Ring (strict)"("Visible"=TRUE) -> ()  [unwired: 2 in, 2 out]
                n169 = property on="Test Slider" class="Slide (strict)"("Visible"=FALSE) -> ()  [unwired: 2 in, 2 out]
              }
              frame "Exposure  **" {
                n170 = Index Array(array=w291, index=2) -> (element=w292:cluster{string[]})
                n171 = call <vilib>:"NT Read String.vi"("Name"=w294) -> ("String"=w293:string)  [unwired: 9 in, 1 out]
                n172 = Unbundle(w292) -> (w288:string[])
                n173 = Match First String(2:w288, 3:w293) -> (0:w289:i32)  [unwired: 1 out]
                n174 = property on="Test Ring" class="Ring (strict)"("Value"=w289, "Strings []"=w288) -> ()  [unwired: 2 in, 2 out]
                n175 = property on="Test Ring" class="Ring (strict)"("Visible"=TRUE) -> ()  [unwired: 2 in, 2 out]
                n176 = property on="Test Slider" class="Slide (strict)"("Visible"=FALSE) -> ()  [unwired: 2 in, 2 out]
              }
              frame "Exposure Priority  **" {
                n177 = Index Array(array=w300, index=3) -> (element=w301:cluster{string[]})
                n178 = call <vilib>:"NT Read String.vi"("Name"=w303) -> ("String"=w302:string)  [unwired: 9 in, 1 out]
                n179 = Unbundle(w301) -> (w297:string[])
                n180 = Match First String(2:w297, 3:w302) -> (0:w298:i32)  [unwired: 1 out]
                n181 = property on="Test Ring" class="Ring (strict)"("Value"=w298, "Strings []"=w297) -> ()  [unwired: 2 in, 2 out]
                n182 = property on="Test Ring" class="Ring (strict)"("Visible"=TRUE) -> ()  [unwired: 2 in, 2 out]
                n183 = property on="Test Slider" class="Slide (strict)"("Visible"=FALSE) -> ()  [unwired: 2 in, 2 out]
              }
              frame "Color Enable  **" {
                n184 = Index Array(array=w309, index=4) -> (element=w310:cluster{string[]})
                n185 = call <vilib>:"NT Read String.vi"("Name"=w312) -> ("String"=w311:string)  [unwired: 9 in, 1 out]
                n186 = Unbundle(w310) -> (w306:string[])
                n187 = Match First String(2:w306, 3:w311) -> (0:w307:i32)  [unwired: 1 out]
                n188 = property on="Test Ring" class="Ring (strict)"("Value"=w307, "Strings []"=w306) -> ()  [unwired: 2 in, 2 out]
                n189 = property on="Test Ring" class="Ring (strict)"("Visible"=TRUE) -> ()  [unwired: 2 in, 2 out]
                n190 = property on="Test Slider" class="Slide (strict)"("Visible"=FALSE) -> ()  [unwired: 2 in, 2 out]
              }
              frame Default {
                n191 = property on="Test Ring" class="Ring (strict)"("Visible"=FALSE) -> ()  [unwired: 2 in, 2 out]
                n192 = property on="Test Slider" class="Slide (strict)"("Visible"=FALSE) -> ()  [unwired: 2 in, 2 out]
              }
              frame "Brightness  **", "Color Level  **", "Compression  **", "FPS  **", "Sharpness  **" {
                n193 = call <vilib>:"NT Read Number.vi"("Name"=w318) -> ("Numeric"=w317:dbl)  [unwired: 9 in, 1 out]
                n194 = local write "Test Slider"(w317) -> ()
                n195 = property on="Test Slider" class="Slide (strict)"("Visible"=TRUE, "Scale.Maximum"=100.0 ("Scale.Range:Maximum")) -> ()  [unwired: 2 in, 2 out]
                n196 = property on="Test Ring" class="Ring (strict)"("Visible"=FALSE) -> ()  [unwired: 2 in, 2 out]
              }
            }
          }
        }
        n197 = property on="Progress" class="Clust (strict)"("Visible"=FALSE) -> ()  [unwired: 2 in, 2 out]
      }
      event "Test Name": Mouse Enter {
        # "Populate the ring with the list of tests"
        n198 = event-data() -> ()  [unwired: 1 in, 1 out]
        n199 = call <vilib>:"NT Read String Array.vi"("Name"="/TestMode/TestList") -> ("String Array"=w327:string[])  [unwired: 9 in, 1 out]
        n200 = Build Array (concatenate)("Select the test to run...", w327) -> (w326:string[])
        n201 = property on="Test Name" class="Ring (strict)"("Strings []"=w326) -> ()  [unwired: 2 in, 2 out]
      }
      event "Test Name": Value Change {
        w330 = FALSE ("Visible")
        # "Tell the robot the test name to run"
        n202 = event-data() -> ("NewVal"=w334:u16)  [unwired: 1 in]
        n203 = property on="Test Name" class="Ring (strict)"() -> ("Strings []"=w335:string[])  [unwired: 2 in, 2 out]
        n204 = local write "Progress"(T7 {"Test Progress"=0, "Test Progress Text"=""} ("Progress")) -> ()
        n205 = Index Array(array=w335, index=w334) -> (element=w333:string)
        n206 = call <vilib>:"NT Write String.vi"("String"=w333, "Name"="/TestMode/TestName") -> ()  [unwired: 9 in, 1 out]
        n207 = property on="Progress" class="Clust (strict)"("Visible"=TRUE) -> ()  [unwired: 2 in, 2 out]
        n208 = property on="Motor" class="Clust (strict)"("Visible"=w330) -> ()  [unwired: 2 in, 2 out]
        n209 = property on="Test Slider" class="Slide (strict)"("Visible"=w330) -> ()  [unwired: 2 in, 2 out]
        n210 = property on="On/Off" class="Bool (strict)"("Visible"=w330) -> ()  [unwired: 2 in, 2 out]
        n211 = property on="Rev/Fwd" class="Clust (strict)"("Visible"=w330) -> ()  [unwired: 2 in, 2 out]
        n212 = property on="Test Ring" class="Ring (strict)"("Visible"=w330) -> ()  [unwired: 2 in, 2 out]
      }
      event "Select Auto": Mouse Enter {
        # "Populate the combo box with the list of autonomous options"
        n213 = event-data() -> ()  [unwired: 1 in, 1 out]
        n214 = call <vilib>:"NT Read String Array.vi"("Name"="Auto List") -> ("String Array"=w337:string[])  [unwired: 9 in, 1 out]
        n215 = property on="Select Auto" class="CmbBox"("Strings[]"=w337) -> ()  [unwired: 2 in, 2 out]
      }
      event "Select Auto": Value Change {
        # "User modified the Auto Selection. Write to NT variable so robot knows."
        n216 = event-data() -> ("NewVal"=w341:string)  [unwired: 1 in]
        n217 = call <vilib>:"NT Write String.vi"("String"=w341, "Name"="Auto Selector") -> ()  [unwired: 9 in, 1 out]
      }
      event "Command Selection": Value Change {
        # "Get the params and show in table"
        n218 = event-data() -> ("NewVal"=w348:i32)  [unwired: 1 in]
        n219 = property on="Command Selection" class="MCListbox (strict)"() -> ("ItemNames"=w346:string[][])  [unwired: 2 in, 2 out]
        n220 = call <vilib>:"WPI_DashboardUpdate Command Params.vi"("NewVal"=w348, "Commands"=w346, "Param Tbl"=w347) -> ()  [unwired: 8 in, 1 out]
      }
      event "Execute Command": Value Change {
        # "Started one, Unique ID holds\nresponse"
        n221 = event-data() -> ()  [unwired: 1 in, 1 out]
        n222 = property on="Command Selection" class="MCListbox (strict)"() -> ("ItemNames"=w360:string[][])  [unwired: 2 in, 2 out]
        n223 = Index Array(array=w360, index (row)="Command Selection", index (col)=0) -> (element=w358:string)
        n224 = call <vilib>:"Invoke Commands.vi"("Command Params"="Command Params", "Function Name"=w358) -> ("Params"=w354:u8, "Started"=w353:bool)  [unwired: 7 in, 1 out]
        n225 = Array Subset(array="Command Params", length (row)=w354) -> (w355:string[][])  [unwired: 3 in]
        n226 = Select(t="Executing" ("Cmd Status"), s=w353, f="" ("Cmd Status")) -> (s? t:f=→"Cmd Status":string)
      }
      event "Command Selection": Double Click {
        n227 = event-data() -> ("Row"=w370:i32)  [unwired: 1 in]
        n228 = property on="Command Selection" class="MCListbox (strict)"() -> ("ItemNames"=w373:string[][])  [unwired: 2 in, 2 out]
        n229 = local read "Command Params"() -> (w368:string[][])
        n230 = Index Array(array=w373, index (row)=w370, index (col)=0) -> (element=w371:string)
        n231 = call <vilib>:"Invoke Commands.vi"("Command Params"=w368, "Function Name"=w371) -> ("Params"=w367:u8, "Started"=w362:bool)  [unwired: 7 in, 1 out]
        n232 = Array Subset(array=w368, length (row)=w367) -> (w366:string[][])  [unwired: 3 in]
        n233 = Select(t="Executing" ("Cmd Status"), s=w362, f="" ("Cmd Status")) -> (s? t:f=w363:string)
        n234 = local write "Cmd Status"(w363) -> ()
      }
      event "CheckList": Double Click {
        # "Shift clears all"
        # "Update symbols on the listbox"
        n235 = event-data() -> ("PlatMods.Shift"=w376:bool, "Row"=w378:i32)  [unwired: 1 in]
        n236 = case shown="True" w376 {
          tunnel: w378 -> [w382 _]
          tunnel: 1 -> [w381 _]
          frame False {
            n237 = property on="CheckList" class="LstBox (strict)"() -> ("Item Symbols"=w380:i32[])  [unwired: 2 in, 2 out]
            n238 = Replace Array Subset(array=w380, new element=w381, index=w382) -> (w379:i32[])
            n239 = property on="CheckList" class="LstBox (strict)"("Item Symbols"=w379) -> ()  [unwired: 2 in, 2 out]
          }
          frame True {
            w383 = 0 ("Top Row")
            n240 = property on="CheckList" class="LstBox (strict)"() -> ("Number of Rows"=w385:u32)  [unwired: 2 in, 2 out]
            n241 = Initialize Array(0, w385) -> (w384:i32[])
            n242 = property on="CheckList" class="LstBox (strict)"("Top Row"=w383, "Value"=w383, "Item Symbols"=w384) -> ()  [unwired: 2 in, 2 out]
          }
        }
      }
      event "CheckList": Key Down {
        # "Update symbols on the listbox\nLeft and right keys check and uncheck"
        n243 = event-data() -> ("VKey"=w390:T22)  [unwired: 1 in]
        n244 = case shown="\"Left\", \"Right\"" w390 {
          selector: w390 -> [w395 _]
          tunnel: eventvkey."Left" ("VKey") -> [w393 _]
          frame "Left", "Right" {
            n245 = Equal?(x=w393, y=w395) -> (x = y?=w394:bool)
            n246 = Select(t=0, s=w394, f=1) -> (s? t:f=w396:i32)
            n247 = property on="CheckList" class="LstBox (strict)"() -> ("Item Symbols"=w399:i32[])  [unwired: 2 in, 2 out]
            n248 = Replace Array Subset(array=w399, new element=w396, index="CheckList") -> (w398:i32[])
            n249 = property on="CheckList" class="LstBox (strict)"("Item Symbols"=w398) -> ()  [unwired: 2 in, 2 out]
          }
          frame Default {
          }
        }
      }
      event "DB Camera Config": Value Change {
        # "Show or hide the cluster of controls, store in ini file"
        n250 = event-data() -> ("NewVal"=w404:bool)  [unwired: 1 in]
        n251 = case shown="False" w404 {
          tunnel: w403 -> [w413 _]
          tunnel: [w406 w424] -> w402
          tunnel: w401 -> [w405 w424]
          frame False {
            w420 = "Camera"
            w423 = FALSE ("Visible")
            n252 = local read "Camera Settings"() -> (w412:T2)
            n253 = Index Array(array=w413) -> (element=w416:cluster{string[]})  [unwired: 1 in]
            n254 = Unbundle(w412) -> ("Frame Rate"=w411:i32, "Compression"=w410:i32, "Size"=w414:u16)
            n255 = Unbundle(w416) -> (w415:string[])
            n256 = Index Array(array=w415, index=w414) -> (element=w409:string)
            n257 = call-poly <vilib>:"Write Key.vi"("section"=w420, "value"=w409, "key"="Size", "refnum"=w405) -> ("refnum out"=w422:T20)  [unwired: 2 in, 5 out]
            n258 = call-poly <vilib>:"Write Key.vi"("section"=w420, "value"=w411, "key"="FrameRate", "refnum"=w422) -> ("refnum out"=w421:T20)  [unwired: 1 in, 6 out]
            n259 = property on="Camera Settings" class="Clust (strict)"("Visible"=w423) -> ()  [unwired: 2 in, 2 out]
            n260 = local write "DB Camera Config"(w423) -> ()
            n261 = call-poly <vilib>:"Write Key.vi"("section"=w420, "value"=w410, "key"="Compression", "refnum"=w421) -> ("refnum out"=w407:T20)  [unwired: 1 in, 6 out]
            n262 = call <vilib>:"Close Config Data.vi"("refnum"=w407) -> ("file path"=w408:path)  [unwired: 2 in, 8 out]
            n263 = call <vilib>:"Open Config Data.vi"("configuration file path"=w408) -> ("refnum"=w406:T20)  [unwired: 8 in, 2 out]
          }
          frame True {
            n264 = property on="Camera Settings" class="Clust (strict)"("Visible"=TRUE) -> ()  [unwired: 2 in, 2 out]
          }
        }
      }
      event "Camera Settings": Value Change {
        # "Update summary string when any elements of DB camera change"
        n265 = event-data() -> ("NewVal"=w438:T2)  [unwired: 1 in]
        n266 = Index Array(array=w434) -> (element=w433:cluster{string[]})  [unwired: 1 in]
        n267 = Unbundle(w438) -> ("Frame Rate"=w429:i32, "Compression"=w428:i32, "Size"=w431:u16)
        n268 = Unbundle(w433) -> (w432:string[])
        n269 = Index Array(array=w432, index=w431) -> (element=w430:string)
        n270 = Format Into String(format string="%s   %dfps   %d%%", w430, w429, w428) -> (resulting string=w435:string)  [unwired: 2 in, 1 out]
        n271 = Build Array(w435) -> (w436:string[])
        n272 = property on="DB Camera Config" class="Bool (strict)"("Strings [4]"=w436) -> ()  [unwired: 2 in, 2 out]
      }
      event "Motor.Enable": Value Change {
        # "When the test mode otor enable helper is set, update that\ntree row item's value"
        n273 = event-data() -> ("NewVal"=w445:bool)  [unwired: 1 in]
        n274 = Unbundle("Motor") -> ("Value"=w444:dbl)  [unwired: 1 out]
        n275 = Select(t=w444, s=w445, f=0.0) -> (s? t:f=w442:dbl)
        n276 = call <vilib>:"NT Write Number.vi"("Numeric"=w442, "Name"=w441) -> ()  [unwired: 9 in, 1 out]
      }
      event "Test Slider": Value Change {
        # "When the test mode slider helper is set, update that\ntree row item's value"
        n277 = event-data() -> ("NewVal"=w449:dbl)  [unwired: 1 in]
        n278 = call <vilib>:"NT Write Number.vi"("Numeric"=w449, "Name"=w450) -> ()  [unwired: 9 in, 1 out]
      }
      event "On/Off": Value Change {
        # "When the test mode on/off helper value is set, update that\ntree row item's value"
        n279 = event-data() -> ("NewVal"=w455:bool)  [unwired: 1 in]
        n280 = Boolean To (0,1)(Boolean=w455) -> (0, 1=w454:i16)
        n281 = call <vilib>:"NT Write Number.vi"("Numeric"=w454, "Name"=w453) -> ()  [unwired: 9 in, 1 out]
      }
      event "Rev/Fwd": Value Change {
        # "When the test mode helper value for relays is set, update that\ntree row item's value"
        n282 = event-data() -> ("NewVal.Forward"=w464:bool, "NewVal.Reverse"=w463:bool)  [unwired: 1 in]
        n283 = Boolean To (0,1)(Boolean=w464) -> (0, 1=w460:i16)
        n284 = Boolean To (0,1)(Boolean=w463) -> (0, 1=w462:i16)
        n285 = Negate(x=w462) -> (-x=w461:i16)
        n286 = Add(x=w460, y=w461) -> (x+y=w459:i16)
        n287 = call <vilib>:"NT Write Number.vi"("Numeric"=w459, "Name"=w458) -> ()  [unwired: 9 in, 1 out]
      }
      event "Test Ring": Value Change {
        # "When a test mode helper value is selected from the ring,\nset the tree item's variable to the string value"
        n288 = event-data() -> ("NewVal"=w469:u16)  [unwired: 1 in]
        n289 = property on="Test Ring" class="Ring (strict)"() -> ("Strings []"=w470:string[])  [unwired: 2 in, 2 out]
        n290 = Index Array(array=w470, index=w469) -> (element=w468:string)
        n291 = call <vilib>:"NT Write String.vi"("String"=w468, "Name"=w467) -> ()  [unwired: 9 in, 1 out]
      }
      event "Rec Mode": Value Change {
        # "Update globals for recording mode and path to read log from.\nClear when logging and let NetworkTables set path for vision to\nuse."
        n292 = event-data() -> ("NewVal"=w482:enum32{"Stop", "Record", "Playback"})  [unwired: 1 in]
        n293 = global write "WPI_DashboardLogging Global.vi" "Logging Filename"(path "") -> ()
        n294 = global write "WPI_DashboardLogging Global.vi" "Recording"(w482) -> ()
        n295 = case shown="\"Playback\"" w482 {
          tunnel: w481 -> [_ w484 w493]
          tunnel: [_ _ w492] -> w478
          tunnel: [_ _ w491] -> _
          tunnel: w476 -> [_ _ w489]
          tunnel: cluster{i32, i32} {-250, 170} -> [_ _ w488]
          tunnel: [_ _ T23 {"Image Size"=TRUE, "Image Type"=TRUE, "Pixel Value"=TRUE, "ROI Information"=TRUE, "Zoom Factor"=FALSE} ("Image Information Shown:All Elements")] -> w474
          tunnel: [_ _ TRUE ("Zoom Factor")] -> w473
          tunnel: w472 -> [_ _ w485]
          frame Default {
          }
          frame "Stop", "Record" {
            # "Place Window too"
            n296 = invoke class="VI" method="FP.Close"(reference=w484) -> (reference out=w483:refnum<vi>)  [unwired: 2 in, 2 out]
            n297 = invoke class="VI" method="Abort VI"(reference=w483) -> ()  [unwired: 2 in, 3 out]
          }
          frame "Playback" {
            n298 = call "Open Playback Panel.vi"("Offset"=w488, "DB VI Ref"=w489, "Playback in"=w493) -> ("Playback out"=w490:refnum<vi>)  [unwired: 8 in]
            n299 = register-events(w490, w485) -> (reference out=w492:refnum<event-registration>, error out=w491:errorcluster)  [unwired: 2 in]
          }
        }
        n300 = property on="Camera Image" class="ImageControl"("Image Information Shown"=w474, "Image Information Visible"=w473) -> ()  [unwired: 2 in, 2 out]
        n301 = call <vilib>:"WPI_DashboardNT Log FieldName Cache.vi"("Operation"=enum16{"Lookup/Add", "Index", "Clear"}."Clear") -> ()  [unwired: 8 in, 3 out]
      }
      event Panel Close {
        w495 = enum32{"Stop", "Record", "Playback"}."Stop" ("Rec Mode")
        # "Playback window has been closed, abort"
        n302 = event-data() -> ()  [unwired: 1 in, 4 out]
        n303 = local write "Rec Mode"(w495) -> ()
        n304 = global write "WPI_DashboardLogging Global.vi" "Recording"(w495) -> ()
      }
      event Panel Close {
        # "Abort playback window and ourself"
        n305 = event-data() -> ()  [unwired: 1 in, 4 out]
        n306 = invoke class="VI" method="FP.Close"(reference=w501) -> (reference out=w500:refnum<vi>)  [unwired: 2 in, 2 out]
        n307 = invoke class="VI" method="Abort VI"(reference=w500) -> (error out=w499:errorcluster)  [unwired: 2 in, 2 out]
        n308 = invoke class="VI" method="Abort VI"(error in=w499) -> ()  [unwired: 2 in, 3 out]
      }
      event User Event {
        n309 = event-data() -> ("IDs"=w509:cluster{"RPC field ID":u16, "Unique ID":u16}, "String"=w508:string)  [unwired: 1 in]
        n310 = Bundle("IDs"=w509, "String"=w508) -> (w507:T9)  [unwired: 1 in]
        n311 = call <vilib>:"Retrieve RPC Response.vi"("RPC Response"=w507) -> ("Output"=w504:string[][])  [unwired: 10 in]
        n312 = Build Array (concatenate)(w502, w504) -> (w503:string[][])
        n313 = local write "Command Params"(w503) -> ()
        n314 = local write "Cmd Status"("" ("Cmd Status")) -> ()
      }
      event "Vision": Value Change {
        # "Enable/Disable Compression slider.\nHW USB is hard-coded into the camera"
        n315 = event-data() -> ("NewVal"=w516:u16)  [unwired: 1 in]
        n316 = Equal?(x=w516, y=u32 2 ("milliseconds to wait")) -> (x = y?=w514:bool)
        n317 = Select(t=T24."Disabled and Grayed Out" ("Disabled"), s=w514, f=T24."Enabled" ("Disabled")) -> (s? t:f=w511:T24)
        n318 = property on="Compression" class="Slide (strict)"("DisabledEnum"=w511) -> ()  [unwired: 2 in, 2 out]
      }
      event "Tree": Double Click {
        n319 = event-data() -> ("PlatMods"=w521:T27, "Tag"=w520:string)  [unwired: 1 in]
        n320 = Unbundle(w521) -> ("Shift"=w519:bool)  [unwired: 4 out]
        n321 = Not(x=w519) -> (.not. x?=w518:bool)
        n322 = call <vilib>:"NT Update Persistence.vi"("Persistence"=w518, "Name"=w520) -> ()  [unwired: 9 in, 1 out]
      }
    }
  }
  n323 = while {
    tunnel: w47 -> [w525]
    i -> [w528]
    stop <- FALSE stop-if-true
    n324 = Wait (ms)(milliseconds to wait=u32 100) -> ()  [unwired: 1 out]
    n325 = case shown="\"Playback\"" "Rec Mode" {
      tunnel: w528 -> [_ _ w543]
      tunnel: [u32 2829099 ("Base Color") u32 11141120 ("Target Color") w532] -> w524
      frame "Stop", Default {
        # "Reset the color, extra updates don't cost much"
      }
      frame "Record" {
      }
      frame "Playback" {
        # "Playback"
        n326 = Quotient & Remainder(x=w543, y=u32 50 ("milliseconds to wait")) -> (x-y*floor(x/y)=w539:u32)  [unwired: 1 out]
        n327 = Divide(x=w539, y=u32 50 ("milliseconds to wait")) -> (x/y=w536:dbl)
        n328 = Multiply(x=6.283185307179586, y=w536) -> (x*y=w541:dbl)
        n329 = Sine(x=w541) -> (sin(x)=w540:dbl)
        n330 = Absolute Value(x=w540) -> (abs(x)=w533:dbl)
        n331 = call "Interpolate RGB Color.vi"("Proportion"=w533, "Target Color"=u32 30976, "Base Color"=u32 2829099) -> ("Result Color"=w532:u32)  [unwired: 8 in]
      }
    }
    n332 = property class="Pane"(reference=w525, "PaneColor"=w524) -> ()  [unwired: 1 in, 2 out]
  }
  n333 = local write "Dashboard Tab"(T1."Drive" ("Dashboard Tab")) -> ()
  n334 = property on="On/Off" class="Bool (strict)"("Visible"=w15) -> ()  [unwired: 2 in, 2 out]
  n335 = property on="Motor" class="Clust (strict)"("Visible"=w15) -> ()  [unwired: 2 in, 2 out]
  n336 = property on="Progress" class="Clust (strict)"("Visible"=w15) -> ()  [unwired: 2 in, 2 out]
  n337 = property on="Test Ring" class="Ring (strict)"("Visible"=w15) -> ()  [unwired: 2 in, 2 out]
  n338 = property on="Rev/Fwd" class="Clust (strict)"("Visible"=w15) -> ()  [unwired: 2 in, 2 out]
  n339 = property on="Camera Settings" class="Clust (strict)"("Visible"=w15) -> ()  [unwired: 2 in, 2 out]
  n340 = local write "DB Camera Config"(w15) -> ()
  n341 = local write "Command Params"(string[][] [] ("Command Params")) -> ()
  n342 = global write "WPI_DashboardLogging Global.vi" "Recording"(w41) -> ()
  n343 = local write "Rec Mode"(w41) -> ()
  n344 = while {
    tunnel: u16 1741 ("timeout ms (25000)") -> [w545]
    stop <- FALSE stop-if-true
    n345 = TCP Create Listener(10:w545) -> (0:w544:errorcluster, 3:w546:refnum<k5>)  [unwired: 4 in, 1 out]
    n346 = case shown="No Error" w544 {
      selector: w544 -> [w548 _]
      tunnel: w546 -> [w549 _]
      frame No Error {
        n347 = while {
          tunnel: w549 -> [w552]
          tunnel: w548 -> [w551]
          stop <- FALSE stop-if-true
          n348 = TCP Wait On Listener(8:w551, 11:w552) -> (0:w553:errorcluster, 4:w554:refnum<k5>)  [unwired: 2 in, 3 out]
          n349 = local write "TCP"(w554) -> ()
          n350 = case shown="No Error" w553 {
            frame No Error {
            }
            frame Error {
              n351 = Wait (ms)(milliseconds to wait=u32 1000) -> ()  [unwired: 1 out]
            }
          }
        }
      }
      frame Error {
        n352 = Wait (ms)(milliseconds to wait=u32 1000) -> ()  [unwired: 1 out]
      }
    }
  }
  n353 = local write "Command Selection"(u16 0 ("milliseconds to wait")) -> ()
